vi "EcrireLireValeurParDefaut_HoloTrackPy_locate.vi"(7 "Lecture/Ecriture":enum32{"Lecture", "Ecriture"}(radio), 8 "error in (no error)":errorcluster, 11 "ParamIN":T1={"PythonVer"="3.10", "Python/Environnement\npath"=path "", "HoloPath"=path "", "HoloDir"=path "", "HoloParam"={"wavelength"=6.6e-07, "optical index"=1.33, "Holo size X"=1024, "Holo size Y"=1024, "pixel size"=7e-06, "objective magnification"=40.0}, "Remove mean Hologram"=TRUE, "propagation"={"distance ini"=0.0, "number of planes"=100, "step"=1e-06}, "Fourier BP filter (pix)"={"High pass (0=none)"=15.0, "Low Pass (0=none)"=125.0}, "Focus"={"Type"=enum."SUM_OF_VARIANCE", "Sum size"=15}, "Batch thresold "=enum."compute on each hologram", "CCL parameters"={"Threshold ( N x Standard deviation)"=10.0, "Connectivity"=enum."26", "min voxel"=3.0, "max voxel"=0.0}} {"HoloParam"."Holo size X" format="%.0g"; "HoloParam"."pixel size" format="%#_6e"; "HoloParam"."wavelength" format="%#_6e"; "CCL parameters"."max voxel" min=0.0 max=0.0; "CCL parameters"."min voxel" min=1.0 max=100.0; "CCL parameters"."Threshold ( N x Standard deviation)" min=1.0 max=100.0}) -> (0 "error out":errorcluster, 1 "OK?":bool, 2 "XML File Path(duplicate)":path, 3 "ParamOUT":T1={"PythonVer"="3.10", "Python/Environnement\npath"=path "", "HoloPath"=path "C:/TRAVAIL/developpement/imagesHolo/1000im_manip3/100um_40x_int_.7ajmvz4e.000000.bmp", "HoloDir"=path "C:/TRAVAIL/developpement/imagesHolo/1000im_manip3", "HoloParam"={"wavelength"=6.6e-07, "optical index"=1.33, "Holo size X"=1024, "Holo size Y"=1024, "pixel size"=7e-06, "objective magnification"=40.0}, "Remove mean Hologram"=TRUE, "propagation"={"distance ini"=0.0, "number of planes"=100, "step"=1e-06}, "Fourier BP filter (pix)"={"High pass (0=none)"=15.0, "Low Pass (0=none)"=125.0}, "Focus"={"Type"=enum."SUM_OF_VARIANCE", "Sum size"=15}, "Batch thresold "=enum."compute on each hologram", "CCL parameters"={"Threshold ( N x Standard deviation)"=2.0, "Connectivity"=enum."18", "min voxel"=0.0, "max voxel"=0.0}} {"HoloParam"."Holo size X" format="%.0g"; "HoloParam"."pixel size" format="%#_6e"; "HoloParam"."wavelength" format="%#_6e"; "CCL parameters"."max voxel" min=0.0 max=0.0; "CCL parameters"."min voxel" min=1.0 max=100.0; "CCL parameters"."Threshold ( N x Standard deviation)" min=1.0 max=100.0})   [LabVIEW 2023]
uses:
  param_defaut.ctl
  HologramInfo.ctl
  HoloPyLib/CCL_parameters.ctl
  <vilib>/Utility/xml.llb/Write to XML File(string).vi
  <vilib>/Utility/xml.llb/Read From XML File(string).vi
  HoloPyLib/holoPyTracks.lvlib
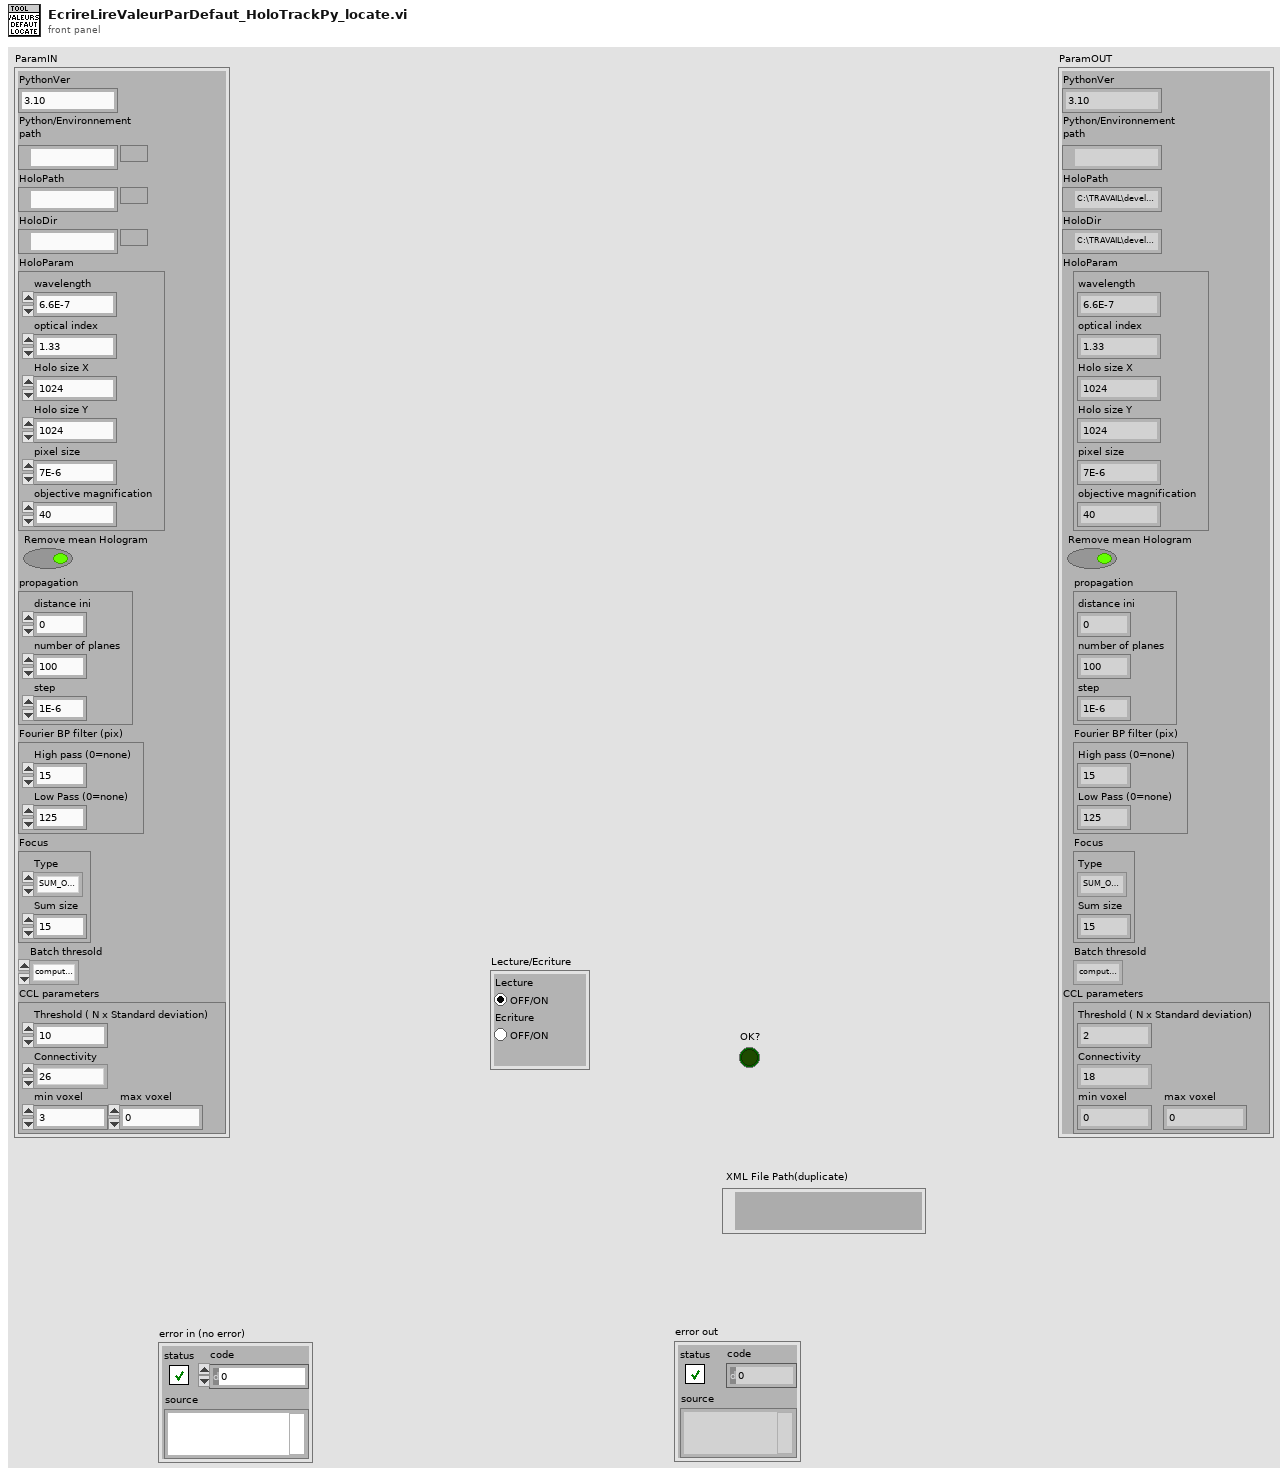
[diagram p1: front panel]
types:
  T1 = typedef "param_defaut.ctl" = cluster{"PythonVer":string, "Python/Environnement\npath":path, "HoloPath":path, "HoloDir":path, "HoloParam":T2, "Remove mean Hologram":bool, "propagation":cluster{"distance ini":dbl, "number of planes":i32, "step":dbl}, "Fourier BP filter (pix)":cluster{"High pass (0=none)":dbl, "Low Pass (0=none)":dbl}, "Focus":cluster{"Type":enum16{"SUM_OF_INTENSITY", "SUM_OF_LAPLACIAN", "SUM_OF_VARIANCE", "TENENGRAD"}, "Sum size":i32}, "Batch thresold ":enum16{"compute on 1st hologram", "compute on each hologram"}, "CCL parameters":T3}
  T2 = typedef "holoPyTracks.lvlib/HologramInfo.ctl" = cluster{"wavelength":sgl, "optical index":sgl, "Holo size X":i32, "Holo size Y":i32, "pixel size":sgl, "objective magnification":sgl}
  T3 = typedef "CCL_parameters.ctl" = cluster{"Threshold ( N x Standard deviation)":dbl, "Connectivity":enum16{"6", "18", "26"}, "min voxel":dbl, "max voxel":dbl}
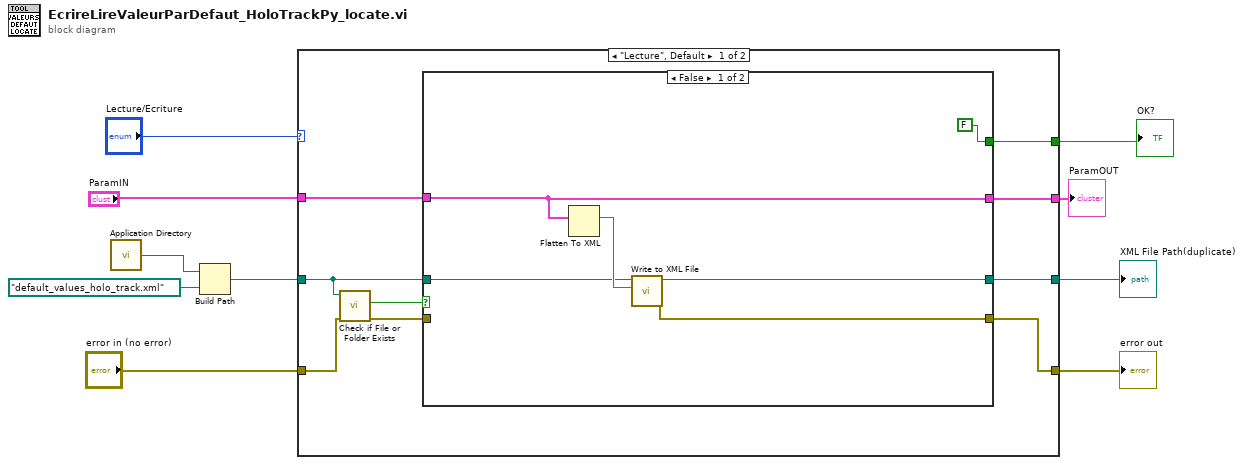
[diagram p0: block diagram]
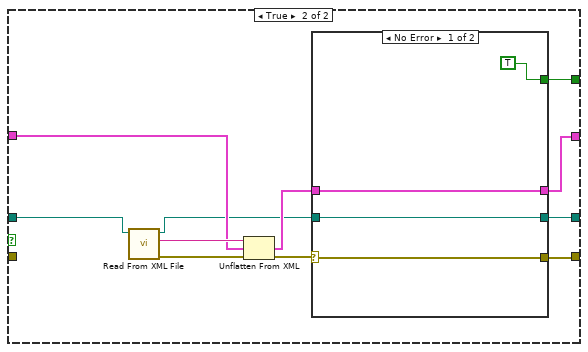
[diagram p2: hidden frame]
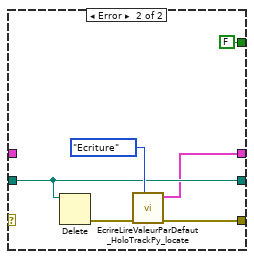
[diagram p3: hidden frame]
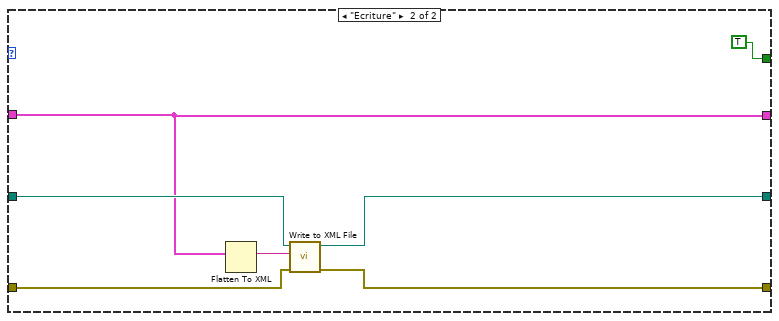
[diagram p4: hidden frame]
diagram:
  n1 = call <vilib>:"Application Directory.vi"() -> ("Application Directory"=w4:path)
  n2 = Build Path(base path=w4, name or relative path=path "default_values_holo_track.xml" ("default name")) -> (appended path=w9:path)
  n3 = case shown="\"Lecture\", Default" "Lecture/Ecriture" {
    tunnel: w9 -> [w17 w52]
    tunnel: "error in (no error)" -> [w16 w51]
    tunnel: [w18 w50] -> w7
    tunnel: [w19 w49] -> w6
    tunnel: "ParamIN" -> [w13 w48]
    tunnel: [w12 w48] -> w1
    tunnel: [w11 TRUE ("OK?")] -> w3
    frame "Lecture", Default {
      n4 = call <vilib>:"Check if File or Folder Exists.vi"("error in (no error)"=w16, "path"=w17) -> ("error out"=w15:errorcluster, "file or folder exists?"=w14:bool)  [unwired: 7 in, 1 out]
      n5 = case shown="False" w14 {
        tunnel: [w21 w30] -> w12
        tunnel: [w22 w27] -> w19
        tunnel: [w24 w31] -> w18
        tunnel: w17 -> [w23 w34]
        tunnel: w15 -> [_ _]
        tunnel: w13 -> [w21 w33]
        tunnel: [FALSE ("OK?") w26] -> w11
        frame False {
          n6 = Flatten To XML(6:w21) -> (2:w25:string)
          n7 = call-poly <vilib>:"Write to XML File.vi"("XML Input"=w25, "XML File Path"=w23) -> ("error out"=w24:errorcluster, "XML File Path(duplicate)"=w22:path)  [unwired: 3 in, 5 out]
        }
        frame True {
          n8 = call-poly <vilib>:"Read From XML File.vi"("XML File Path"=w34) -> ("error out"=w36:errorcluster, "XML Elements"=w35:string, "XML File Path(duplicate)"=w28:path)  [unwired: 8 in]
          n9 = Unflatten From XML(xml string=w35, type=w33, error in (no error)=w36) -> (value=w29:T1, error out=w32:errorcluster)
          n10 = case shown="No Error" w32 {
            selector: w32 -> [w40 _]
            tunnel: [w40 w44] -> w31
            tunnel: [w39 w41] -> w30
            tunnel: w29 -> [w39 _]
            tunnel: w28 -> [w38 w43]
            tunnel: [w38 w43] -> w27
            tunnel: [TRUE ("OK?") FALSE ("OK?")] -> w26
            frame No Error {
            }
            frame Error {
              n11 = Delete(path (use dialog)=w43) -> (error out=w46:errorcluster)  [unwired: 4 in, 2 out]
              n12 = call "EcrireLireValeurParDefaut_HoloTrackPy_locate.vi"("Lecture/Ecriture"=enum32{"Lecture", "Ecriture"}."Ecriture", "error in (no error)"=w46) -> ("error out"=w44:errorcluster, "ParamOUT"=w41:T1)  [unwired: 6 in, 2 out]
            }
          }
        }
      }
    }
    frame "Ecriture" {
      n13 = Flatten To XML(6:w48) -> (2:w53:string)
      n14 = call-poly <vilib>:"Write to XML File.vi"("error in (no error)"=w51, "XML Input"=w53, "XML File Path"=w52) -> ("error out"=w50:errorcluster, "XML File Path(duplicate)"=w49:path)  [unwired: 2 in, 5 out]
    }
  }
  "error out" <- w7
  "XML File Path(duplicate)" <- w6
  "OK?" <- w3
  "ParamOUT" <- w1
